vi "gen_ref.vi"(2 "error in (no error)":errorcluster, 3 "T":dbl, 4 "N":i32) -> (0 "error out":errorcluster, 1 "w_ref":dbl[][][](array[numeric]))   [LabVIEW 2021]
uses:
  <vilib>/Analysis/Matrix/Datatypes/RealMatrix.ctl
  <vilib>/Analysis/Matrix/NI_Matrix.lvlib
panel:
  out "xkp1":T1
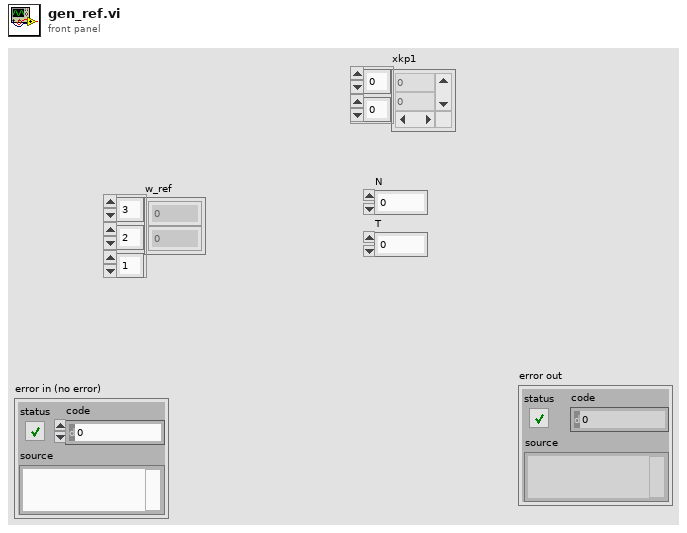
[diagram p1: front panel]
types:
  T1 = typedef "NI_Matrix.lvlib/RealMatrix.ctl" = dbl[][]
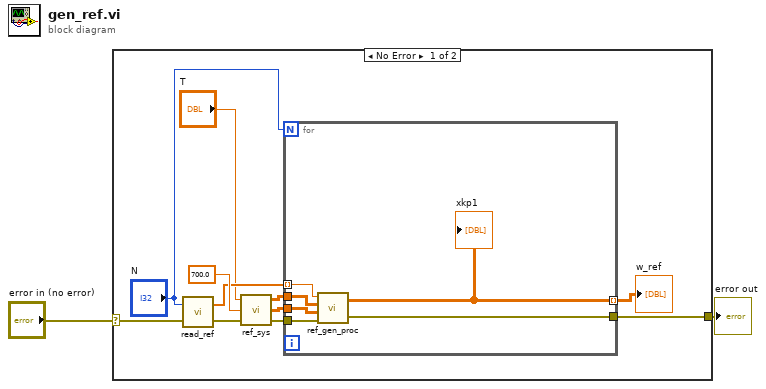
[diagram p0: block diagram]
diagram:
  n1 = case shown="No Error" "error in (no error)" {
    selector: "error in (no error)" -> [w13 w20]
    tunnel: [w6 w20] -> w1
    frame No Error {
      n2 = call "read_ref.vi"("error in (no error)"=w13, "N"="N") -> ("error out"=w10:errorcluster, "wd"=w7:dbl[])
      n3 = call "ref_sys.vi"("error in (no error)"=w10, "wr"=700.0, "T"="T") -> ("error out"=w8:errorcluster, "B"=w12:T1, "A"=w11:T1)
      n4 = for {
        N: "N" -> [_]
        tunnel: w8 -> [w19]
        tunnel: w12 -> [w18]
        tunnel: w11 -> [w17]
        tunnel: w7 -> [w16] mode=indexing
        tunnel: [w15] -> w6
        tunnel: [w14] -> w3 mode=indexing
        n5 = call "ref_gen_proc.vi"("error in (no error)"=w19, "B"=w18, "A"=w17, "wd"=w16) -> ("error out"=w15:errorcluster, "xkp1"=w14:T1)
        "xkp1" <- w14
      }
      "w_ref" <- w3
    }
    frame Error {
    }
  }
  "error out" <- w1
